vi "Controlador Humitat Q_N2.vi"(2 "Humidity setpoint (%RH)":sgl=48.0, 3 "Humidity (%RH)":sgl) -> (0 "Q N2 setpoint (l/min)":sgl)   [LabVIEW 2015, in "VIPM2.lvlib"]
doc: "Control del flux de nitrògen per baixar la humitat.\nControlador P amb saturació a un tram.\nInclou els paràmetres de sintonització."
uses:
  VIPM2.lvlib
panel:
  out "HumiError (%RH)":sgl
  # "Controlador P amb saturació a un tram"
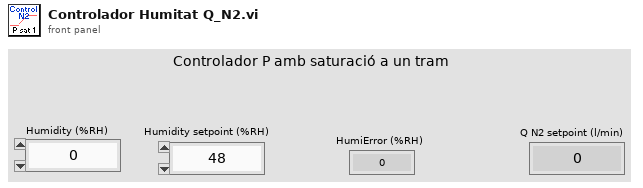
[diagram p1: front panel]
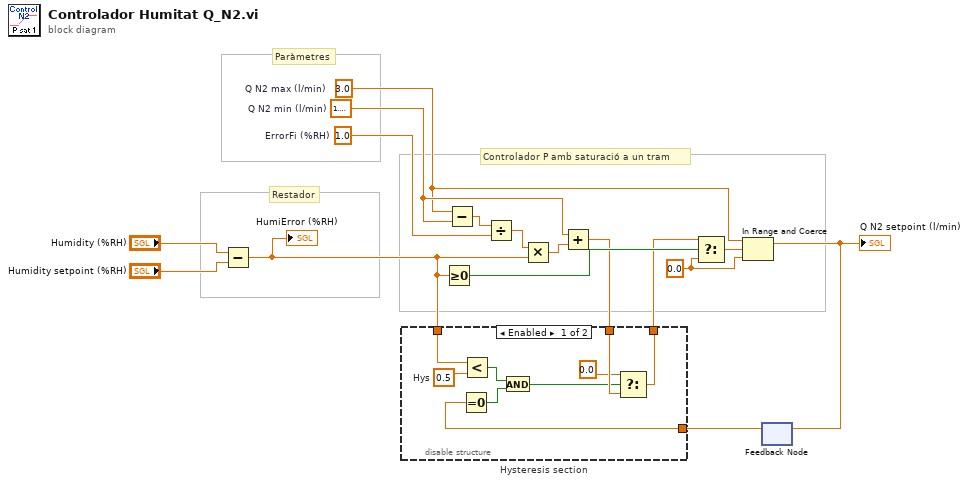
[diagram p0: block diagram]
diagram:
  w7 = sgl 0.0 ("lower limit")
  w13 = sgl 1.0  # ErrorFi (%RH)
  w10 = sgl 1.3  # Q N2 min (l/min)
  w9 = sgl 3.0  # Q N2 max (l/min)
  # "Controlador P amb saturació a un tram"
  # "Restador"
  # "Paràmetres"
  n1 = Subtract(x="Humidity (%RH)", y="Humidity setpoint (%RH)") -> (x-y=w5:sgl)
  "HumiError (%RH)" <- w5
  n2 = Greater Or Equal To 0?(x=w5) -> (x >= 0?=w4:bool)
  n3 = Subtract(x=w9, y=w10) -> (x-y=w14:sgl)
  n4 = Divide(x=w14, y=w13) -> (x/y=w12:sgl)
  n5 = Multiply(x=w12, y=w5) -> (x*y=w11:sgl)
  n6 = Add(x=w10, y=w11) -> (x+y=w2:sgl)
  n7 = feedback #1() -> (w1:sgl)  [unwired: 1 in]
  n8 = disable-structure "Hysteresis section" shown="Enabled" {
    disable-tunnel: w5 -> [w25 _]
    disable-tunnel: [w24 w26] -> w3
    disable-tunnel: w2 -> [w23 w26]
    disable-tunnel: w1 -> [w21 _]
    frame Enabled {
      w22 = sgl 0.5  # Hys
      n9 = Equal To 0?(x=w21) -> (x = 0?=w20:bool)
      n10 = Less?(x=w25, y=w22) -> (x < y?=w19:bool)
      n11 = And(x=w19, y=w20) -> (x .and. y?=w18:bool)
      n12 = Select(t=sgl 0.0, s=w18, f=w23) -> (s? t:f=w24:sgl)
    }
    frame Disabled {
    }
  }
  n13 = Select(t=w3, s=w4, f=w7) -> (s? t:f=w8:sgl)
  n14 = In Range and Coerce(upper limit=w9, x=w8, lower limit=w7) -> (coerced(x)=w6:sgl)  [unwired: 1 out]
  "Q N2 setpoint (l/min)" <- w6
  n15 = feedback-in #1(w6) -> ()
